vi "ExSubStartExpPulser.vi"(2 "error in (no error)":errorcluster, 3 "Handles In":T1) -> (0 "error out":errorcluster, 1 "Handles Out":T1)   [LabVIEW 2010]
panel:
  # "ExSubStartExpPulser:\nThis is a sub-vI that starts the camera and the\nPTG pulser for data collection."
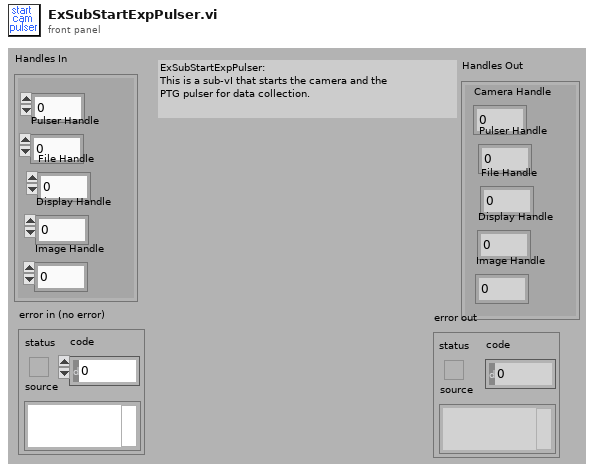
[diagram p1: front panel]
types:
  T1 = cluster{"Camera Handle":u32, "Pulser Handle":u32, "File Handle":u32, "Display Handle":u32, "Image Handle":u32}
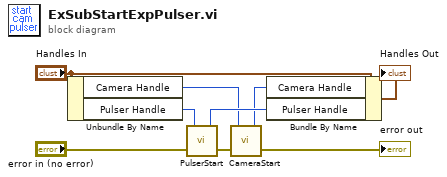
[diagram p0: block diagram]
diagram:
  n1 = Unbundle By Name("Handles In") -> ("Camera Handle"=w2:u32, "Pulser Handle"=w4:u32)
  n2 = call <userlib>:"PulserStart.vi"("error in (no error)"="error in (no error)", "Pulser Handle"=w4) -> ("error out"=w8:errorcluster, "Pulser Handle"=w3:u32)
  n3 = call <userlib>:"CameraStart.vi"("error in"=w8, "Camera Handle"=w2) -> ("error out"=→"error out":errorcluster, "Camera Handle"=w1:u32)
  n4 = Bundle By Name(cluster="Handles In", "Camera Handle"=w1, "Pulser Handle"=w3) -> (→"Handles Out":T1)
